vi "start.vi"(8 "error in (no error)":errorcluster, 11 "SignalReaderCN091129DAQmx in":refnum<class "SignalReaderCN091129DAQmx.lvclass">) -> (0 "error out":errorcluster, 3 "SignalReaderCN091129DAQmx out":refnum<class "SignalReaderCN091129DAQmx.lvclass">)   [LabVIEW 2010, in "SignalReaderCN091129DAQmx.lvclass"]
uses:
  SignalReaderCN091129DAQmx.lvclass
  GenericSignalReader/GenericSignalReader/GenericSignalReader.lvclass
  SignalReaderCN091129DAQmx.lvclass/SignalReaderCN091129DAQmx.ctl
  <vilib>/DAQmx/configure/timing.llb/DAQmx Timing (Sample Clock).vi
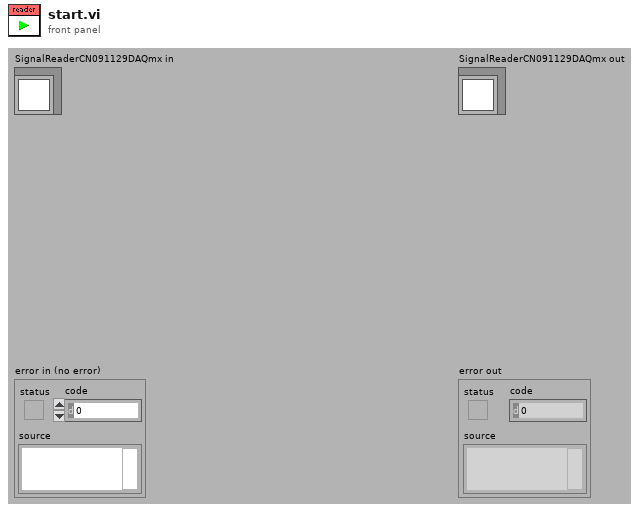
[diagram p1: front panel]
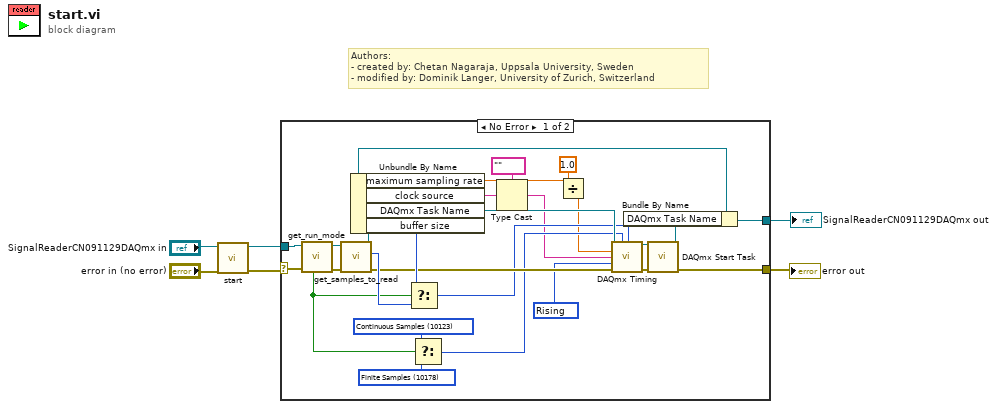
[diagram p0: block diagram]
diagram:
  # "Authors: \n- created by: Chetan Nagaraja, Uppsala University, Sweden\n- modified by: Dominik Langer, University of Zurich, Switzerland"
  n1 = call-parent "start.vi"("error in (no error)"="error in (no error)", "GenericSignalReader in"="SignalReaderCN091129DAQmx in") -> ("error out"=w4:errorcluster, "GenericSignalReader out"=w3:refnum<class "SignalReaderCN091129DAQmx.lvclass">)  [unwired: 8 in]
  n2 = case shown="No Error" w4 {
    selector: w4 -> [w25 w33]
    tunnel: w3 -> [w21 w34]
    tunnel: [w23 w34] -> w2
    tunnel: [w22 w33] -> w1
    frame No Error {
      w13 = 10280 items=["Rising"=10280, "Falling"=10171] ("active edge")
      w29 = 10123 items=["Finite Samples"=10178, "Continuous Samples"=10123, "Hardware Timed Single Point"=12522] ("sample mode")
      w28 = 10178 items=["Finite Samples"=10178, "Continuous Samples"=10123, "Hardware Timed Single Point"=12522] ("sample mode")
      n3 = call-dynamic "get_run_mode.vi"("error in (no error)"=w25, "GenericPlugin in"=w21) -> ("error out"=w26:errorcluster, "GenericPlugin out"=w27:refnum<class "SignalReaderCN091129DAQmx.lvclass">, "is free run?"=w31:bool)  [unwired: 5 in, 2 out]
      n4 = call-dynamic "get_samples_to_read.vi"("error in (no error)"=w26, "GenericSignalReader in"=w27) -> ("error out"=w19:errorcluster, "total samples to read"=w32:i32, "GenericSignalReader out"=w24:refnum<class "SignalReaderCN091129DAQmx.lvclass">)  [unwired: 5 in, 2 out]
      n5 = Unbundle By Name(w24) -> ("maximum sampling rate"=w7:dbl[unit], "clock source"=w8:string, "DAQmx Task Name"=w17:refnum<k21>, "buffer size"=w30:i32)
      n6 = Select(t=w30, s=w31, f=w32) -> (s? t:f=w14:i32)
      n7 = Select(t=w29, s=w31, f=w28) -> (s? t:f=w15:i32)
      n8 = Type Cast(type=tag "" ("source"), x=w8) -> (*(type *) &x=w9:tag)
      n9 = Divide(x=w7, y=dbl[unit] 1.0) -> (x/y=w10:dbl)
      n10 = call-poly <vilib>:"DAQmx Timing.vi"("task/channels in"=w17, "sample mode"=w15, "samples per channel"=w14, "rate"=w10, "source"=w9, "active edge"=w13, "error in"=w19) -> ("task out"=w16:refnum<k21>, "error out"=w18:errorcluster)  [unwired: 7 in]
      n11 = call <vilib>:"DAQmx Start Task.vi"("task/channels in"=w16, "error in"=w18) -> ("task out"=w20:refnum<k21>, "error out"=w22:errorcluster)  [unwired: 12 in]
      n12 = Bundle By Name(cluster=w24, "DAQmx Task Name"=w20) -> (w23:refnum<class "SignalReaderCN091129DAQmx.lvclass">)
    }
    frame Error {
    }
  }
  "error out" <- w1
  "SignalReaderCN091129DAQmx out" <- w2
